vi "虚拟放射源能谱设置.vi"(2 "错误输入（无错误）":errorcluster, 3 "低位数据路径":path, 4 "高位数据路径":path, 5 "VISA资源名称":refnum<visa-resource-name>) -> (0 "错误输出":errorcluster, 1 "VISA资源名称输出":refnum<visa-resource-name>)   [LabVIEW 2014]
uses:
  <vilib>/Utility/file.llb/Read From Spreadsheet File (I64).vi
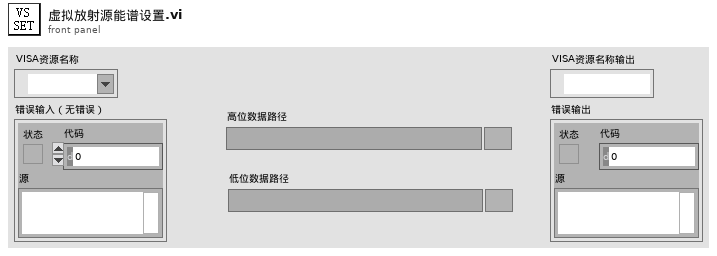
[diagram p1: front panel]
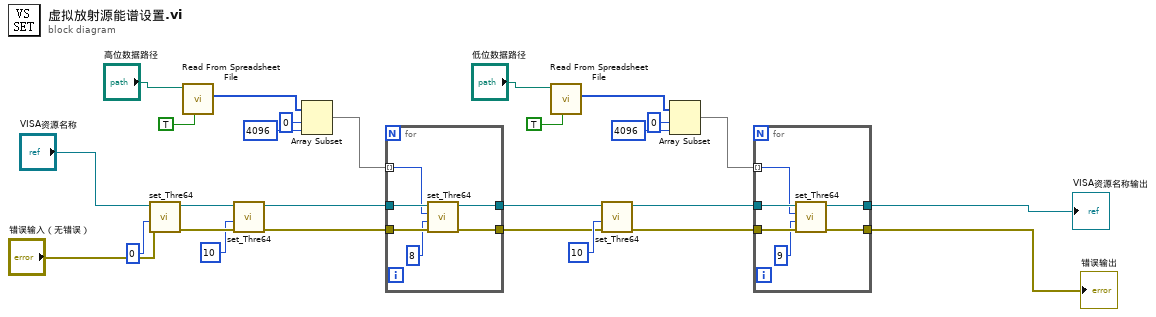
[diagram p0: block diagram]
diagram:
  n1 = call "set_Thre64.vi"("错误输入（无错误）"="错误输入（无错误）", "命令"=u8 0, "VISA资源名称"="VISA资源名称") -> ("错误输出"=w20:errorcluster, "VISA资源名称输出"=w21:refnum<visa-resource-name>)  [unwired: 7 in]
  n2 = call-poly <vilib>:"Read From Spreadsheet File.vi"("transpose (no:F)"=TRUE, "file path (dialog if empty)"="高位数据路径") -> ("first row"=w25:i64[])  [unwired: 5 in, 4 out]
  n3 = call "set_Thre64.vi"("错误输入（无错误）"=w20, "命令"=u8 10, "VISA资源名称"=w21) -> ("错误输出"=w16:errorcluster, "VISA资源名称输出"=w17:refnum<visa-resource-name>)  [unwired: 7 in]
  n4 = Array Subset(array=w25, index=0 ("索引"), length=4096 ("长度")) -> (w18:i64[])
  n5 = for {
    tunnel: w18 -> [w31] mode=indexing
    tunnel: w17 -> [w33]
    tunnel: w16 -> [w32]
    tunnel: [w29] -> w6
    tunnel: [w28] -> w5
    n6 = call "set_Thre64.vi"("错误输入（无错误）"=w32, "命令"=u8 8, "数字"=w31, "VISA资源名称"=w33) -> ("错误输出"=w29:errorcluster, "VISA资源名称输出"=w28:refnum<visa-resource-name>)  [unwired: 6 in]
  }
  n7 = call-poly <vilib>:"Read From Spreadsheet File.vi"("transpose (no:F)"=TRUE, "file path (dialog if empty)"="低位数据路径") -> ("first row"=w9:i64[])  [unwired: 5 in, 4 out]
  n8 = call "set_Thre64.vi"("错误输入（无错误）"=w6, "命令"=u8 10, "VISA资源名称"=w5) -> ("错误输出"=w15:errorcluster, "VISA资源名称输出"=w14:refnum<visa-resource-name>)  [unwired: 7 in]
  n9 = Array Subset(array=w9, index=0 ("索引"), length=4096 ("长度")) -> (w13:i64[])
  n10 = for {
    tunnel: w13 -> [w37] mode=indexing
    tunnel: w14 -> [w39]
    tunnel: w15 -> [w38]
    tunnel: [w35] -> w2
    tunnel: [w34] -> w1
    n11 = call "set_Thre64.vi"("错误输入（无错误）"=w38, "命令"=u8 9, "数字"=w37, "VISA资源名称"=w39) -> ("错误输出"=w34:errorcluster, "VISA资源名称输出"=w35:refnum<visa-resource-name>)  [unwired: 6 in]
  }
  "VISA资源名称输出" <- w2
  "错误输出" <- w1
